vi "lab3.vi"() -> ()   [LabVIEW 2020]
panel:
  in  "Array 2":string[](array[string])
  in  "Array":string[](array[string])
  in  "text":string
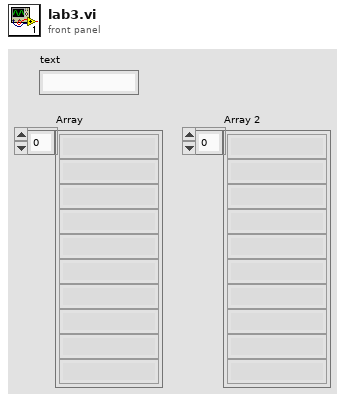
[diagram p1: front panel]
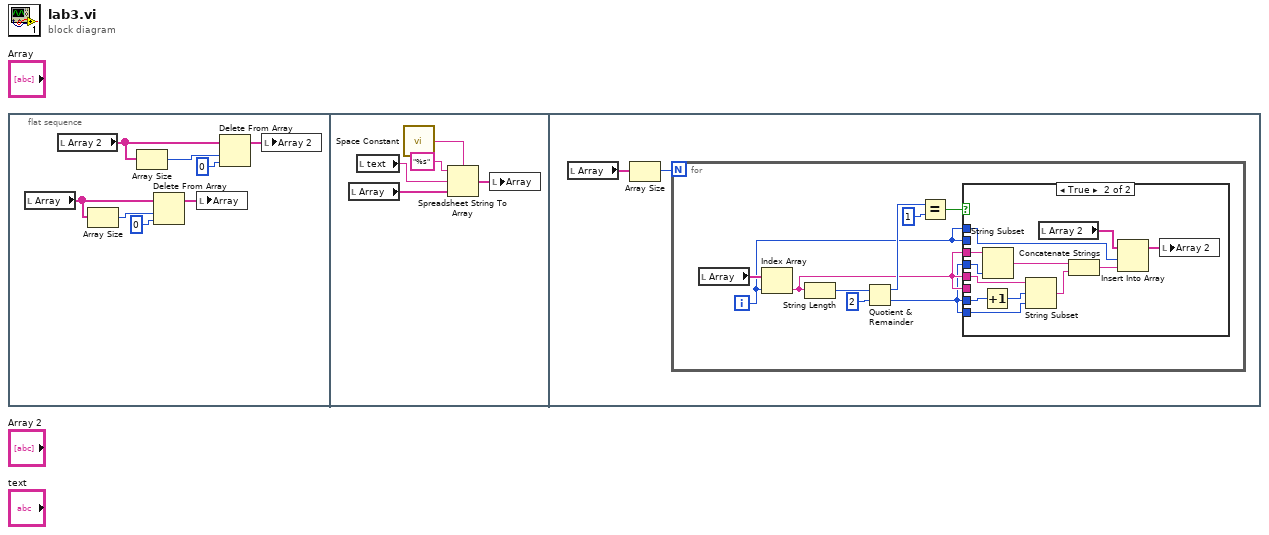
[diagram p0: block diagram]
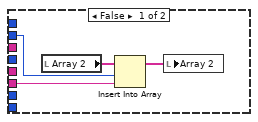
[diagram p2: hidden frame]
diagram:
  n1 = flat-sequence {
    frame #0 {
      n2 = local read "Array"() -> (w6:string[])
      n3 = local read "Array 2"() -> (w2:string[])
      n4 = Array Size(array=w6) -> (size(s)=w8:i32)
      n5 = Array Size(array=w2) -> (size(s)=w4:i32)
      n6 = Delete From Array(array=w6, length=w8, index=0) -> (array with subset deleted=w5:string[])  [unwired: 1 out]
      n7 = local write "Array"(w5) -> ()
      n8 = Delete From Array(array=w2, length=w4, index=0) -> (array with subset deleted=w1:string[])  [unwired: 1 out]
      n9 = local write "Array 2"(w1) -> ()
    }
    frame #1 {
      n10 = local read "Array"() -> (w10:string[])
      n11 = local read "text"() -> (w11:string)
      n12 = call <vilib>:"Space Constant.vi"() -> ("String"=w13:string)
      n13 = Spreadsheet String To Array(delimiter (Tab)=w13, format string="%s", spreadsheet string=w11, array type (2D Dbl)=w10) -> (array=w9:string[])
      n14 = local write "Array"(w9) -> ()
    }
    frame #2 {
      n15 = local read "Array"() -> (w15:string[])
      n16 = Array Size(array=w15) -> (size(s)=w14:i32)
      n17 = for {
        N: w14 -> [_]
        i -> [w16]
        n18 = local read "Array"() -> (w24:string[])
        n19 = Index Array(array=w24, index=w16) -> (element=w18:string)
        n20 = String Length(string=w18) -> (length=w23:i32)
        n21 = Quotient & Remainder(x=w23, y=2) -> (x-y*floor(x/y)=w20:i32, floor(x/y)=w17:i32)
        n22 = Equal?(x=w20, y=1) -> (x = y?=w21:bool)
        n23 = case shown="True" w21 {
          tunnel: w16 -> [w27 _]
          tunnel: w18 -> [w26 _]
          tunnel: w17 -> [_ w40]
          tunnel: w18 -> [_ w39]
          tunnel: w18 -> [_ w38]
          tunnel: w17 -> [_ w37]
          tunnel: w17 -> [_ w35]
          tunnel: w16 -> [_ w31]
          frame False {
            n24 = local read "Array 2"() -> (w28:string[])
            n25 = Insert Into Array(array=w28, index=w27, new element=w26) -> (w25:string[])
            n26 = local write "Array 2"(w25) -> ()
          }
          frame True {
            n27 = Increment(x=w37) -> (x+1=w36:i32)
            n28 = String Subset(string=w39, length (rest)=w40) -> (substring=w34:string)  [unwired: 1 in]
            n29 = String Subset(string=w38, offset (0)=w36, length (rest)=w35) -> (substring=w33:string)
            n30 = local read "Array 2"() -> (w32:string[])
            n31 = Concatenate Strings(w34, w33) -> (w30:string)
            n32 = Insert Into Array(array=w32, index=w31, new element=w30) -> (w29:string[])
            n33 = local write "Array 2"(w29) -> ()
          }
        }
      }
    }
  }
